vi "Write Status.vi"(8 "error in (no error)":errorcluster, 10 "Fore Optics Contents":T1, 11 "Fore Optics in":refnum<class "Fore Optics.lvclass">) -> (0 "error out":errorcluster, 3 "Fore Optics out":refnum<class "Fore Optics.lvclass">)   [LabVIEW 2018, in "Fore Optics.lvclass"]
uses:
  Fore Optics.lvclass
  Fore Optics.lvclass/Fore Optics.ctl
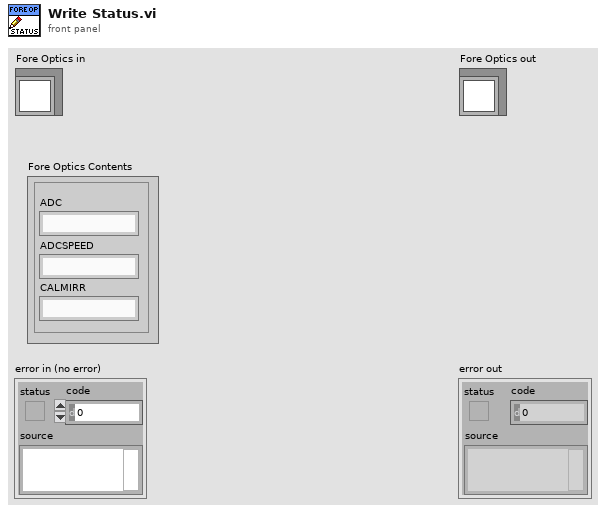
[diagram p1: front panel]
types:
  T1 = cluster{"ADC":string, "ADCSPEED":string, "CALMIRR":string}
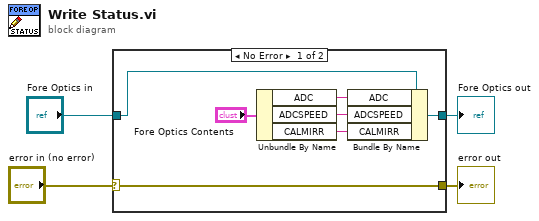
[diagram p0: block diagram]
diagram:
  n1 = case shown="No Error" "error in (no error)" {
    selector: "error in (no error)" -> [w11 w13]
    tunnel: [w11 w13] -> w3
    tunnel: [w9 w12] -> w1
    tunnel: "Fore Optics in" -> [w10 w12]
    frame No Error {
      n2 = Unbundle By Name("Fore Optics Contents") -> ("ADC"=w5:string, "ADCSPEED"=w6:string, "CALMIRR"=w7:string)
      n3 = Bundle By Name(cluster=w10, "ADC"=w5, "ADCSPEED"=w6, "CALMIRR"=w7) -> (w9:refnum<class "Fore Optics.lvclass">)
    }
    frame Error {
    }
  }
  "error out" <- w3
  "Fore Optics out" <- w1
